vi "Create.vi"(6 "Labels":map{string, string}(c390), 7 "Registry Name":string="_default_registry", 8 "error in (no error)":errorcluster, 9 "Auto-register?":bool=TRUE, 10 "Description":string, 11 "Metric Name":string) -> (0 "error out":errorcluster, 3 "Counter Ref":refnum<data-value>)   [LabVIEW 2020, in "Metrics.lvlib" / "Counter.lvclass"]
uses:
  Counter.lvclass
  C:/Github-locals/PromVIEW/src/metrics/metric/Metric.lvclass
  metric/Metric.lvclass/Metric.ctl
  metric/Write Name.vi
  metric/Write Description.vi
  registry/session/Registry Session.lvclass
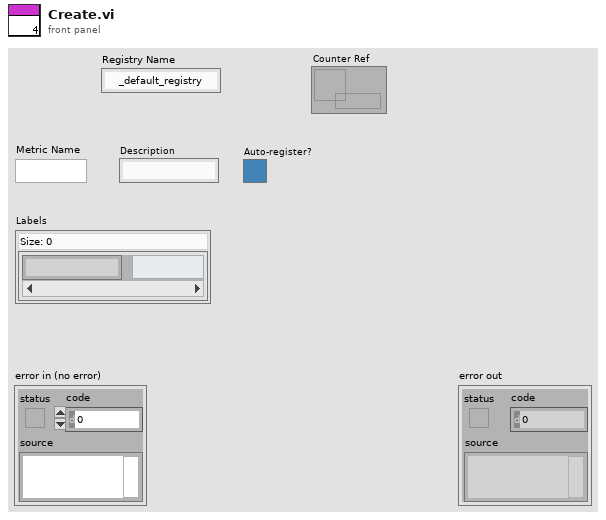
[diagram p1: front panel]
types:
  T1 = enum16{"seconds", "milliseconds", "microseconds"}
  T2 = typedef "Registry.lvlib/Registry Session.lvclass/Session Handle.ctl" = refnum<data-value>
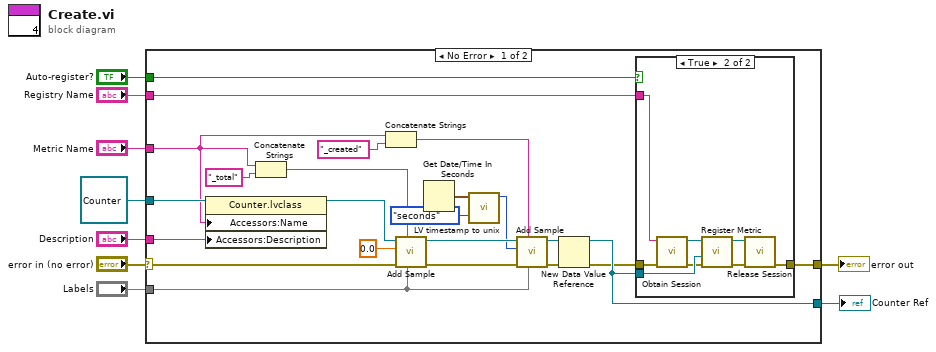
[diagram p0: block diagram]
diagram:
  n1 = case shown="No Error" "error in (no error)" {
    selector: "error in (no error)" -> [w25 w42]
    tunnel: [w17 w42] -> w8
    tunnel: "Metric Name" -> [w16 _]
    tunnel: "Labels" -> [w20 _]
    tunnel: "Description" -> [w29 _]
    tunnel: refnum<class "Counter.lvclass"> refnum ("Metrics.lvlib:Counter.lvclass") -> [w30 _]
    tunnel: [w15 _] -> w3
    tunnel: "Registry Name" -> [w18 _]
    tunnel: "Auto-register?" -> [w13 _]
    frame No Error {
      n2 = property class="Counter.lvclass"(reference=w30, "Accessors:Name"=w16, "Accessors:Description"=w29) -> (reference out=w28:refnum<class "Counter.lvclass">)  [unwired: 1 in, 1 out]
      n3 = Concatenate Strings(w16, "_total" ("string")) -> (w26:string)
      n4 = Concatenate Strings(w16, "_created" ("string")) -> (w19:string)
      n5 = call-dynamic "Add Sample.vi"("Labels"=w20, "Sample Name"=w26, "error in (no error)"=w25, "Value"=0.0, "Metric in"=w28) -> ("error out"=w23:errorcluster, "Metric out"=w24:refnum<class "Counter.lvclass">)  [unwired: 5 in]
      n6 = Get Date/Time In Seconds() -> (seconds since 1Jan1904=w12:timestamp)
      n7 = call "LV timestamp to unix.vi"("Precision (ms)"=T1."seconds", "Timestamp"=w12) -> ("Unix epoch time"=w11:u64)  [unwired: 9 in]
      n8 = call-dynamic "Add Sample.vi"("Labels"=w20, "Sample Name"=w19, "error in (no error)"=w23, "Value"=w11, "Metric in"=w24) -> ("error out"=w21:errorcluster, "Metric out"=w22:refnum<class "Counter.lvclass">)  [unwired: 5 in]
      n9 = New Data Value Reference(data value=w22, error in=w21) -> (data value reference=w15:refnum<data-value>, error out=w14:errorcluster)
      n10 = case shown="True" w13 {
        tunnel: w18 -> [_ w41]
        tunnel: [w33 w35] -> w17
        tunnel: w15 -> [_ w40]
        tunnel: w14 -> [w33 w38]
        frame False {
        }
        frame True {
          n11 = call "Obtain Session.vi"("error in (no error)"=w38, "Session  Name ()"=w41) -> ("error out"=w37:errorcluster, "Session Handle"=w39:T2)  [unwired: 8 in]
          n12 = call "Register Metric.vi"("error in (no error)"=w37, "New Metric"=w40, "Session Handle in"=w39) -> ("error out"=w36:errorcluster, "Session Handle out"=w34:T2)  [unwired: 7 in]
          n13 = call "Release Session.vi"("error in (no error)"=w36, "Session Handle"=w34) -> ("error out"=w35:errorcluster)  [unwired: 9 in]
        }
      }
    }
    frame Error {
    }
  }
  "error out" <- w8
  "Counter Ref" <- w3
